vi "NanotecSMCPD.destructor.vi"(0 "i ref in":refnum<vi>, 5 "error in (no error)":errorcluster) -> (19 "error out":errorcluster)   [LabVIEW 2014, in "NanotecSMCPD.lvlib"]
doc: "This is the destructor of a class.\n\nLicense Agreement for this software:\n\nCopyright (C)\nGesellschaft für Schwerionenforschung, GSI\nPlanckstr. 1\n64291 Darmstadt\nGermany\n\nContact: D.Beck@gsi.de \n\nThis program is free software; you can redistribute it and/or modify it under the terms of the \nGNU General Public License as published by the Free Software Foundation; either version 2 of \nthe license, or (at your option) any later version.\n\nThis program is distributed in the hope that it will be useful, but WITHOUT ANY WARRANTY; \nwithout even the implied warranty of MERCHANTABILITY or FITNESS FOR A PARTICULAR PURPOSE. See the GNU General License for more details (http://www.gnu.org).\n\nGesellschaft für Schwerionenforschung, GSI\nPlanckstr. 1, 64291 Darmstadt, Germany\nFor all questions and ideas contact: M.Richter@gsi.de, H.Brand@gsi.de or D.Beck@gsi.de.\nLast update: 16-JUN-2004"
uses:
  NanotecSMCPD.lvlib
  CSCore/CSApplicationBaseClasses/MotorBase/MotorBase.lvlib
  CSlibraries-extern/DimLVEvent/LVDimInterface/LVDimInterface.lvlib
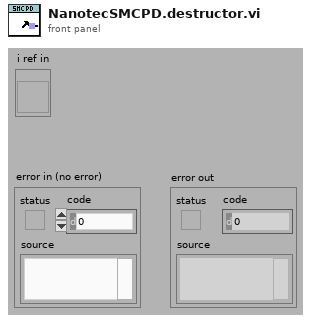
[diagram p1: front panel]
types:
  T1 = typedef "NanotecSMCPD.lvlib/NanotecSMCPD.i attribute.ctl" = cluster{"referencing":bool[], "stop":bool[], "AutoHalt ID":i32, "MethodQueue":refnum<queue>, "Referenced1Time?":bool[], "LastCommand ID":i32}
  T2 = enum16{"SetAttribute", "GetAttribute", "CreateAttribute", "DestroyAttribute", "DestroyAllAtributes"}
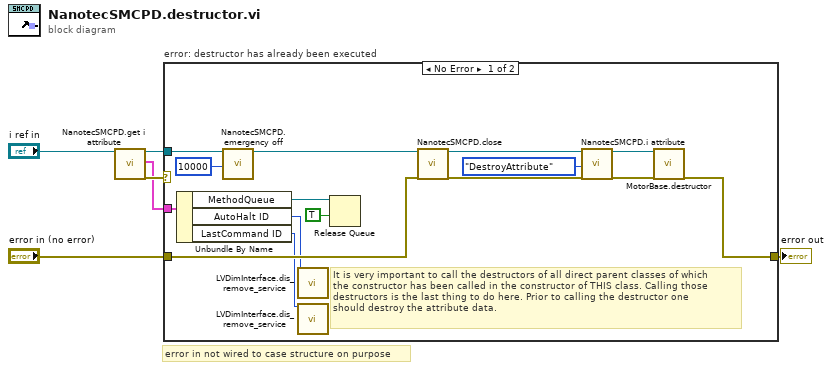
[diagram p0: block diagram]
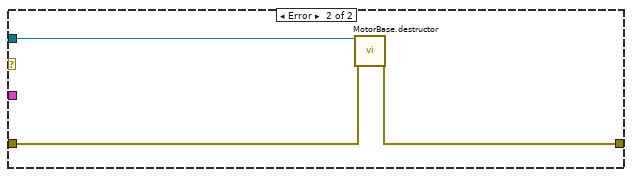
[diagram p2: hidden frame]
diagram:
  # "error in not wired to case structure on purpose"
  n1 = call "NanotecSMCPD.get i attribute.vi"("i ref in"="i ref in") -> ("i ref out"=w2:refnum<vi>, "i attribute"=w1:T1, "error out"=w3:errorcluster)  [unwired: 16 in]
  n2 = case "error: destructor has already been executed" shown="No Error" w3 {
    tunnel: [w18 w22] -> w6
    tunnel: "error in (no error)" -> [w12 w23]
    tunnel: w2 -> [w17 w24]
    tunnel: w1 -> [w11 _]
    frame No Error {
      # "It is very important to call the destructors of all direct parent classes of which\nthe constructor has been called in the constructor of THIS class. Calling those\ndestructors is the last thing to do here. Prior to calling the destructor one \nshould destroy the attribute data."
      n3 = Unbundle By Name(w11) -> ("MethodQueue"=w10:refnum<queue>, "AutoHalt ID"=w8:i32, "LastCommand ID"=w7:i32)
      n4 = call "NanotecSMCPD.emergency off.vi"("i ref in"=w17, "ms timeout (10000)"=10000) -> ("i ref out"=w15:refnum<vi>)  [unwired: 15 in, 2 out]
      n5 = call "LVDimInterface.dis_remove_service.vi"("my_serviceID"=w8) -> ()  [unwired: 18 in, 1 out]
      n6 = call "LVDimInterface.dis_remove_service.vi"("my_serviceID"=w7) -> ()  [unwired: 18 in, 1 out]
      n7 = Release Queue(queue=w10, force destroy? (F)=TRUE) -> ()  [unwired: 1 in, 3 out]
      n8 = call "NanotecSMCPD.close.vi"("i ref in"=w15, "error in (no error)"=w12) -> ("i ref out"=w14:refnum<vi>, "error out"=w13:errorcluster)  [unwired: 16 in]
      n9 = call "NanotecSMCPD.i attribute.vi"("VI Refnum"=w14, "Action"=T2."DestroyAttribute", "error in (no error)"=w13) -> ("VI Refnum out"=w20:refnum<vi>, "error out"=w19:errorcluster)  [unwired: 14 in, 1 out]
      n10 = call "MotorBase.destructor.vi"("i ref in"=w20, "error in (no error)"=w19) -> ("error out"=w18:errorcluster)  [unwired: 17 in]
    }
    frame Error {
      n11 = call "MotorBase.destructor.vi"("i ref in"=w24, "error in (no error)"=w23) -> ("error out"=w22:errorcluster)  [unwired: 17 in]
    }
  }
  "error out" <- w6
